vi "getReminder.vi"(8 "divider":u8=4, 9 "power":i8=-2, 11 "input":u32=4294967294) -> (2 "reminder":u32)   [LabVIEW 2016]
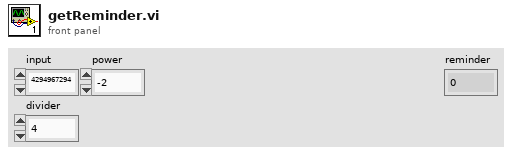
[diagram p1: front panel]
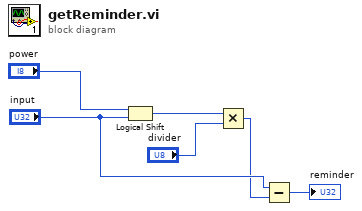
[diagram p0: block diagram]
diagram:
  n1 = Logical Shift(y="power", x="input") -> (x << y=w6:u32)
  n2 = Multiply(x=w6, y="divider") -> (x*y=w4:u32)
  n3 = Subtract(x="input", y=w4) -> (x-y=→"reminder":u32)
